vi "Timeout.vi"(2 "Timeout":dbl, 8 "RST":bool, 9 "Auto RST":bool=TRUE) -> (11 "dT":dbl, 16 "Done":bool=TRUE)   [LabVIEW 2023, in "SFC.lvlib"]
uses:
  SFC.lvlib
panel:
  out "Saved Time":dbl
  out "Init":bool=TRUE
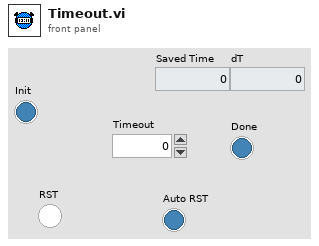
[diagram p1: front panel]
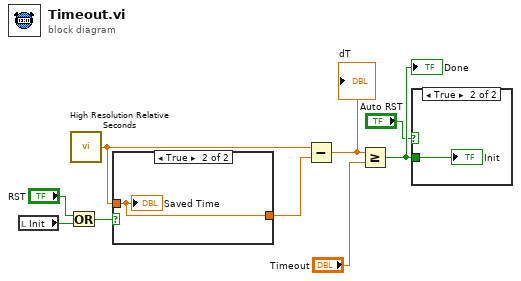
[diagram p0: block diagram]
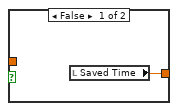
[diagram p3: hidden frame]
diagram:
  n1 = local read "Init"() -> (w9:bool)
  n2 = Or(x="RST", y=w9) -> (x .or. y?=w3:bool)
  n3 = call <vilib>:"High Resolution Relative Seconds.vi"() -> ("relative seconds"=w8:dbl)
  n4 = case shown="True" w3 {
    tunnel: w8 -> [_ w11]
    tunnel: [w10 w11] -> w7
    frame False {
      n5 = local read "Saved Time"() -> (w10:dbl)
    }
    frame True {
      "Saved Time" <- w11
    }
  }
  n6 = Subtract(x=w8, y=w7) -> (x-y=w6:dbl)
  "dT" <- w6
  n7 = Greater Or Equal?(x=w6, y="Timeout") -> (x >= y?=w4:bool)
  "Done" <- w4
  n8 = case shown="True" "Auto RST" {
    tunnel: w4 -> [_ w12]
    frame False {
    }
    frame True {
      "Init" <- w12
    }
  }
